vi "Teleop.vi"(10 "Match Info":T1={"Autonomous Elapsed Seconds"=0.0, "TeleOp Elapsed Seconds"=0.0, "Disabled Elapsed Seconds"=0.0, "Visited Autonomous"=FALSE, "Visited TeleOp"=FALSE, "Visited Disabled"=FALSE, "Autonomous Settings"={"Autonomous Style"=enum."Independent", "VI Refnum"=refnum}}, 11 "Call Context":T2) -> ()   [LabVIEW 2019]
doc: "This VI is called for each TeleOp packet received from the DS where the robot is not disabled. It is often used to read from the joysticks and update I/O or to update setpoints for timed control loops. It should complete and return within 20 milliseconds or it may miss DS packets."
uses:
  <vilib>/Rock Robotics/WPI/DriverStation/WPI_DriverStationDerivedRobotMode.ctl
  <vilib>/Rock Robotics/WPI/DriverStation/WPI_DriverStationMatch Info.ctl
  <vilib>/Rock Robotics/WPI/Utilities/WPI_GetSetVariantRefNum.vi
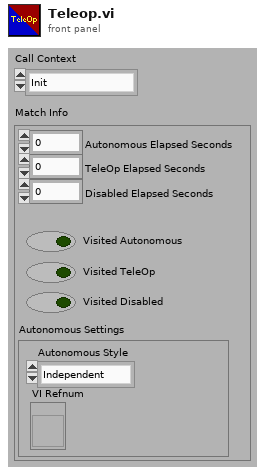
[diagram p1: front panel]
types:
  T1 = typedef "WPI_DriverStationMatch Info.ctl" = cluster{"Autonomous Elapsed Seconds":dbl, "TeleOp Elapsed Seconds":dbl, "Disabled Elapsed Seconds":dbl, "Visited Autonomous":bool, "Visited TeleOp":bool, "Visited Disabled":bool, "Autonomous Settings":cluster{"Autonomous Style":enum16{"Iterative", "Independent"}, "VI Refnum":refnum<vi>}}
  T2 = typedef "WPI_DriverStationDerivedRobotMode.ctl" = enum16{"Init", "Execute", "Stop"}
  T3 = typedef "WPI_JoystickDevRef.ctl" = cluster{"Device":T4}
  T4 = typedef "WPI_JoystickDeviceEnum.ctl" = enum16{"USB 0", "USB 1", "USB 2", "USB 3", "USB 4", "USB 5"}
  T5 = typedef "WPI_RobotDriveDevRef.ctl" = cluster{"DevStatus":errorcluster, "Motors[]":T6[], "Square Inputs":bool, "Max Output":dbl}
  T6 = typedef "WPI_MotorControlDeviceRef.ctl" = cluster{"DeviceStatus":errorcluster, "Type":T7, "PWM":cluster{"PWM Channel":T8, "DeadBand":T9}, "CAN":cluster{"Device Number":u8, "SetOutput VI Ref":variant, "GetOutput VI Ref":variant, "Enable VI Ref":variant, "Disable VI Ref":variant, "Data":variant}, "Invert":bool, "DIO PWM":cluster{"PWM \"Enable\" Channel":T8, "DIOChannel":T10, "PWM Rate":dbl}}
  T7 = typedef "WPI_MotorControlType.ctl" = enum16{"PWM", "CAN", "DIO PWM"}
  T8 = typedef "FPGA_DIOPWMChannel.ctl" = enum8{"PWM 0", "PWM 1", "PWM 2", "PWM 3", "PWM 4", "PWM 5", "PWM 6", "PWM 7", "PWM 8", "PWM 9", "PWM MXP 0", "PWM MXP 1", "PWM MXP 2", "PWM MXP 3", "PWM MXP 4", "PWM MXP 5", "PWM MXP 6", "PWM MXP 7", "PWM MXP 8", "PWM MXP 9", "Invalid"}
  T9 = typedef "WPI_PWMDeadband.ctl" = cluster{"Name":string, "maxPositivePwm":i32, "minPositivePwm":i32, "centerPwm":i32, "maxNegativePwm":i32, "minNegativePwm":i32, "angularRange":u16}
  T10 = typedef "FPGA_DIOChannel.ctl" = enum8{"DIO 0", "DIO 1", "DIO 2", "DIO 3", "DIO 4", "DIO 5", "DIO 6", "DIO 7", "DIO 8", "DIO 9", "DIO MXP 0", "DIO MXP 1", "DIO MXP 2", "DIO MXP 3", "DIO MXP 4", "DIO MXP 5", "DIO MXP 6", "DIO MXP 7", "DIO MXP 8", "DIO MXP 9", "DIO MXP 10", "DIO MXP 11", "DIO MXP 12", "DIO MXP 13", "DIO MXP 14", "DIO MXP 15", "SPI Port CS1", "SPI Port CS2", "SPI Port CS3", "SPI Port MISO", "SPI Port MOSI", "Invalid"}
  T11 = cluster{"JoystickDevRef":T3, "RobotDriveDevRef":T5}
  T12 = typedef "WPI_ServoDeviceRef.ctl" = cluster{"DeviceStatus":errorcluster, "PWM Channel":T8, "DeadBand":T9}
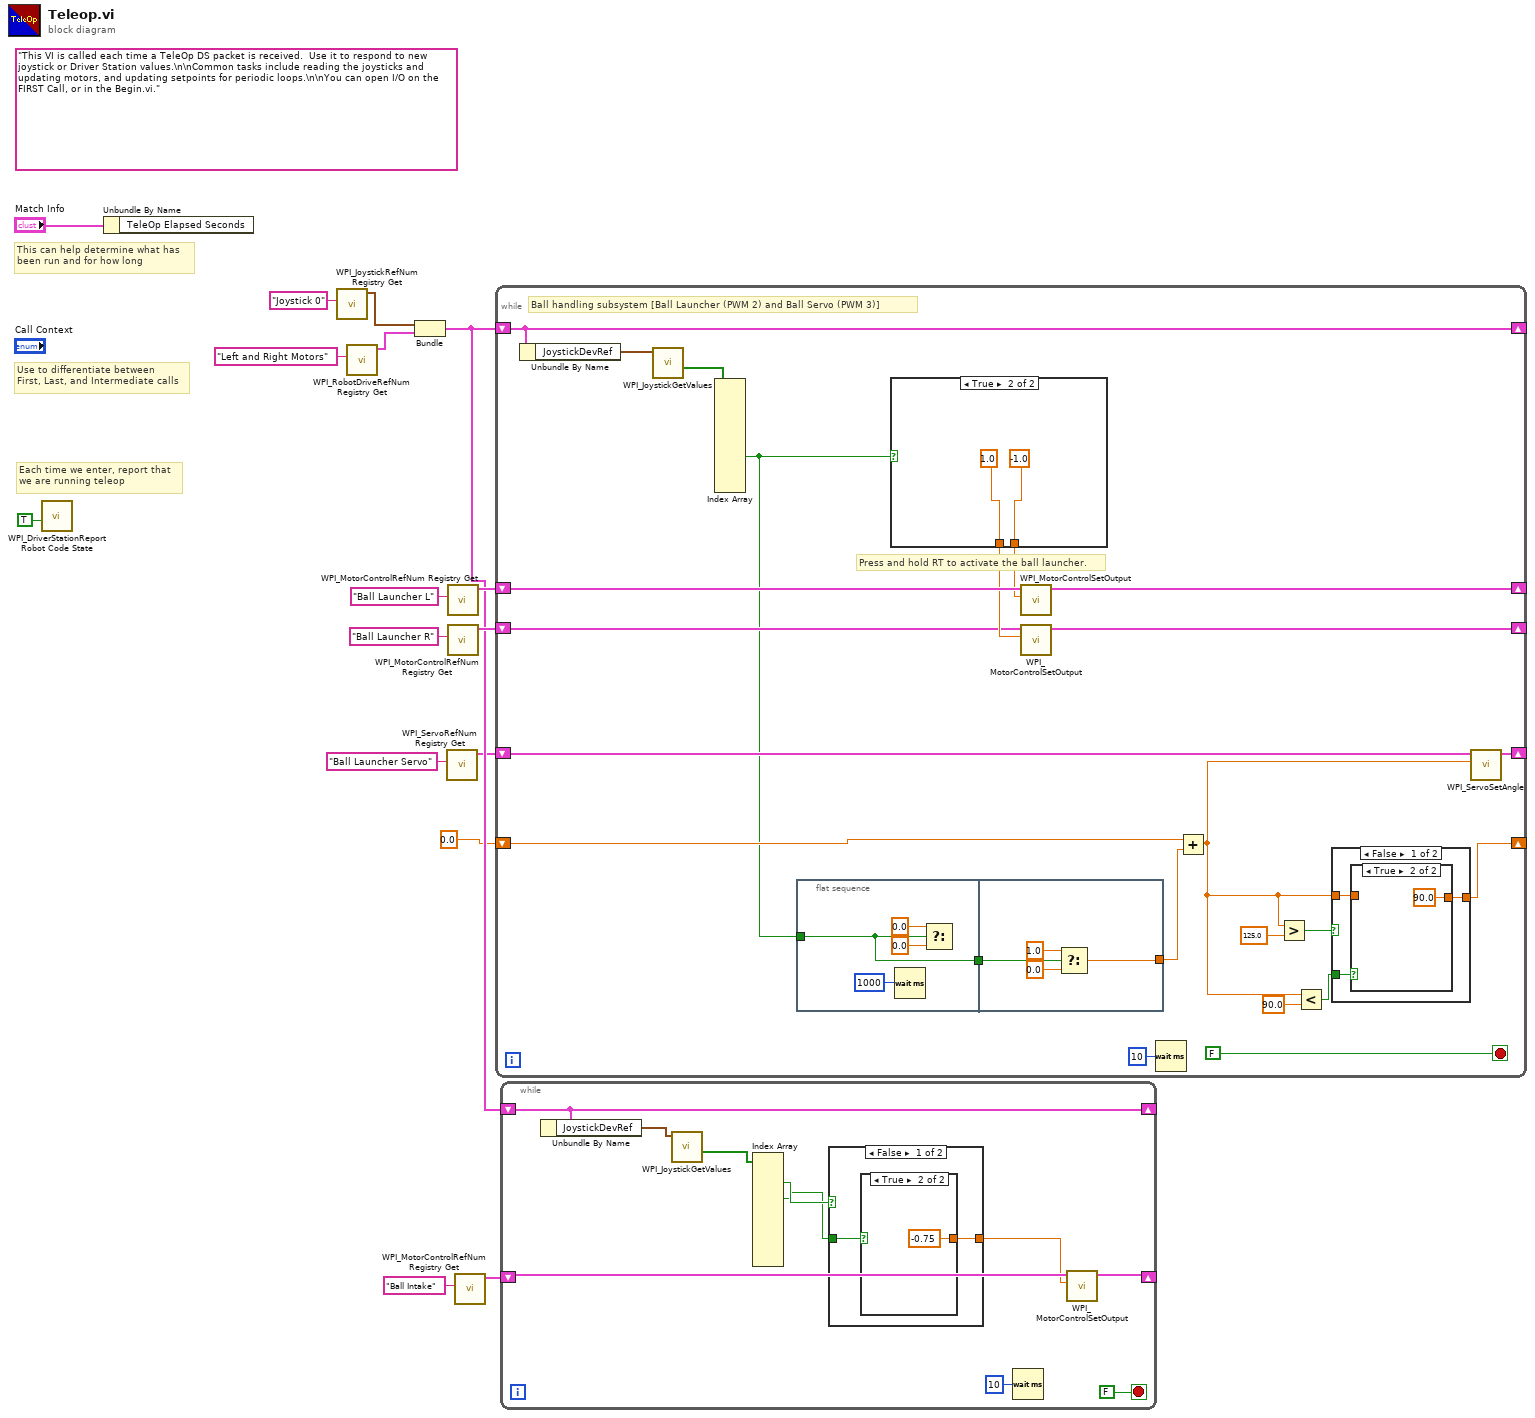
[diagram p0: block diagram]
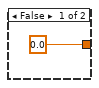
[diagram p2: hidden frame]
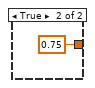
[diagram p3: hidden frame]
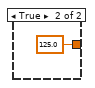
[diagram p5: hidden frame]
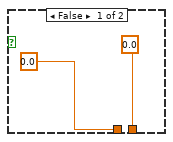
[diagram p6: hidden frame]
diagram:
  (unwired) "This VI is called each time a TeleOp DS packet is received.  Use it to respond to new joystick or Driver Station values.\n\nCommon tasks include reading the joysticks and updating motors, and updating setpoints for periodic loops.\n\nYou can open I/O on the FIRST Call, or in the Begin.vi."
  # "Each time we enter, report that\nwe are running teleop"
  # "Use to differentiate between\nFirst, Last, and Intermediate calls"
  # "This can help determine what has\nbeen run and for how long"
  n1 = call <vilib>:"WPI_DriverStationReport Robot Code State.vi"("TeleOp"=TRUE ("Autonomous")) -> ()  [unwired: 10 in, 1 out]
  n2 = Unbundle By Name("Match Info") -> ()  [unwired: 1 out]
  n3 = call <vilib>:"WPI_JoystickRefNum Registry Get.vi"("refnum name"="Joystick 0") -> ("JoystickDevRef"=w11:T3)  [unwired: 9 in, 1 out]
  n4 = call <vilib>:"WPI_RobotDriveRefNum Registry Get.vi"("refnum name"="Left and Right Motors") -> ("RobotDriveDevRef"=w12:T5)  [unwired: 9 in, 1 out]
  n5 = Bundle("JoystickDevRef"=w11, "RobotDriveDevRef"=w12) -> (w4:T11)  [unwired: 1 in]
  n6 = call <vilib>:"WPI_ServoRefNum Registry Get.vi"("refnum name"="Ball Launcher Servo") -> ("ServoDeviceRef"=w3:T12)  [unwired: 9 in, 1 out]
  n7 = call <vilib>:"WPI_MotorControlRefNum Registry Get.vi"("refnum name"="Ball Launcher L") -> ("MotorControlDevRef"=w10:T6)  [unwired: 9 in, 1 out]
  n8 = call <vilib>:"WPI_MotorControlRefNum Registry Get.vi"("refnum name"="Ball Launcher R") -> ("MotorControlDevRef"=w7:T6)  [unwired: 9 in, 1 out]
  n9 = call <vilib>:"WPI_MotorControlRefNum Registry Get.vi"("refnum name"="Ball Intake") -> ("MotorControlDevRef"=w5:T6)  [unwired: 9 in, 1 out]
  n10 = while {
    shift-right: [w38] -> _
    shift-left: w4 -> [w38]
    shift-right: [w34] -> _
    shift-left: w10 -> [w35]
    shift-right: [w31] -> _
    shift-left: w7 -> [w29]
    shift-right: [w27] -> _
    shift-left: w3 -> [w28]
    shift-right: [w17] -> _
    shift-left: 0.0 ("x") -> [w26]
    stop <- FALSE stop-if-true
    # "Ball handling subsystem [Ball Launcher (PWM 2) and Ball Servo (PWM 3)]"
    # "Press and hold RT to activate the ball launcher."
    n11 = Unbundle By Name(w38) -> ("JoystickDevRef"=w37:T3)
    n12 = call <vilib>:"WPI_JoystickGetValues.vi"("JoystickDevRef"=w37) -> ("Buttons"=w36:bool[])  [unwired: 6 in, 4 out]
    n13 = Index Array(array=w36) -> (element #8=w25:bool)  [unwired: 12 in, 11 out]
    n14 = flat-sequence {
      tunnel: w25 -> [w47]
      tunnel: [w47] -> w24
      tunnel: w24 -> [w53]
      tunnel: [w52] -> w23
      frame #0 {
        n15 = Wait (ms)(milliseconds to wait=u32 1000) -> ()  [unwired: 1 out]
        n16 = Select(t=0.0, s=w47, f=0.0) -> ()  [unwired: 1 out]
      }
      frame #1 {
        n17 = Select(t=1.0, s=w53, f=0.0) -> (s? t:f=w52:dbl)
      }
    }
    n18 = case shown="True" w25 {
      tunnel: [0.0 ("Output") -1.0 ("Output")] -> w33
      tunnel: [0.0 ("Output") 1.0 ("Output")] -> w30
      frame False {
      }
      frame True {
      }
    }
    n19 = call <vilib>:"WPI_MotorControlSetOutput.vi"("Output"=w33, "MotorControlDevRef"=w35) -> ("MotorControlDevRef"=w34:T6)  [unwired: 7 in, 2 out]
    n20 = call <vilib>:"WPI_MotorControlSetOutput.vi"("Output"=w30, "MotorControlDevRef"=w29) -> ("MotorControlDevRef"=w31:T6)  [unwired: 7 in, 2 out]
    n21 = Wait (ms)(milliseconds to wait=u32 10) -> ()  [unwired: 1 out]
    n22 = Add(x=w26, y=w23) -> (x+y=w18:dbl)
    n23 = Greater?(x=w18, y=125.0) -> (0:w21:bool)
    n24 = Less?(x=w18, y=90.0) -> (x < y?=w19:bool)
    n25 = case shown="False" w21 {
      tunnel: w19 -> [w42 _]
      tunnel: w18 -> [w41 _]
      tunnel: [w40 125.0] -> w17
      frame False {
        n26 = case shown="True" w42 {
          tunnel: [w43 90.0] -> w40
          tunnel: w41 -> [w43 _]
          frame False {
          }
          frame True {
          }
        }
      }
      frame True {
      }
    }
    n27 = call <vilib>:"WPI_ServoSetAngle.vi"("Angle"=w18, "ServoDeviceRef"=w28) -> ("ServoDeviceRef"=w27:T12)  [unwired: 8 in, 1 out]
  }
  n28 = while {
    shift-right: [w63] -> _
    shift-left: w5 -> [w62]
    shift-right: [w67] -> _
    shift-left: w4 -> [w67]
    stop <- FALSE stop-if-true
    n29 = Unbundle By Name(w67) -> ("JoystickDevRef"=w66:T3)
    n30 = call <vilib>:"WPI_JoystickGetValues.vi"("JoystickDevRef"=w66) -> ("Buttons"=w65:bool[])  [unwired: 6 in, 4 out]
    n31 = Index Array(array=w65) -> (element #2=w64:bool, element #4=w60:bool)  [unwired: 12 in, 10 out]
    n32 = case shown="False" w64 {
      tunnel: [w69 0.75 ("Output")] -> w61
      tunnel: w60 -> [w68 _]
      frame False {
        n33 = case shown="True" w68 {
          tunnel: [0.0 ("Output") -0.75 ("Output")] -> w69
          frame False {
          }
          frame True {
          }
        }
      }
      frame True {
      }
    }
    n34 = Wait (ms)(milliseconds to wait=u32 10) -> ()  [unwired: 1 out]
    n35 = call <vilib>:"WPI_MotorControlSetOutput.vi"("Output"=w61, "MotorControlDevRef"=w62) -> ("MotorControlDevRef"=w63:T6)  [unwired: 7 in, 2 out]
  }
